vi "ConditionalUnsigned8.vi"(11 "?":u8) -> (2 "Value String":string, 3 "Stop?":bool)   [LabVIEW 2017]
doc: "Displays the value of the 8-bit unsigned integer numeric control and allows conditional breakpoints."
panel:
  in  "Tab Control":enum32{"Data   ", "Condition      "}(tab)
  out "Value":u8
  in  "Ls":u8
  in  "Gr":u8
  in  "Eq":u8
  in  "Ls":bool
  in  "Gr":bool
  in  "Eq":bool
  # "Pause if any of the following:"
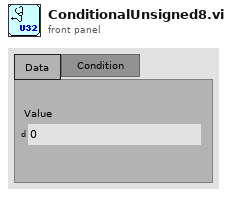
[diagram p1: front panel]
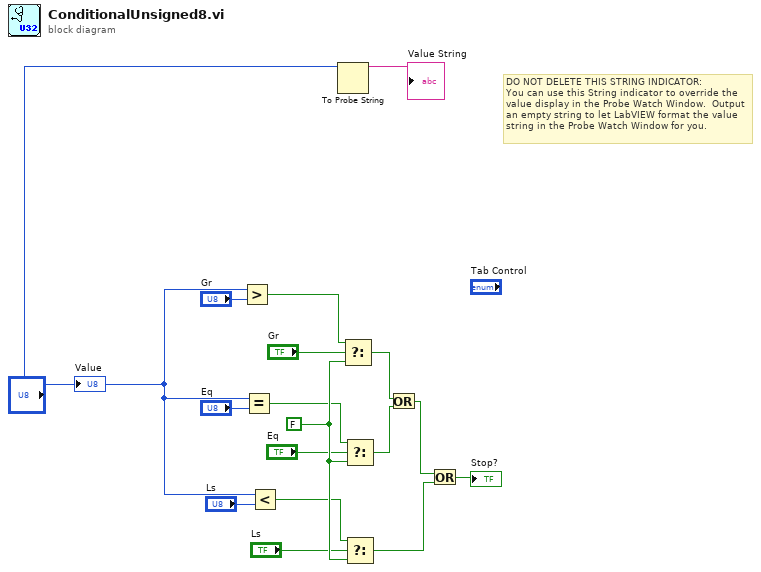
[diagram p0: block diagram]
diagram:
  w14 = FALSE ("f")
  # "DO NOT DELETE THIS STRING INDICATOR: \nYou can use this String indicator to override the value display in the Probe Watch Window.  Output an empty string to let LabVIEW format the value string in the Probe Watch Window for you."
  n1 = Greater?(x="?", y="Gr") -> (0:w2:bool)
  n2 = Equal?(x="?", y="Eq") -> (x = y?=w11:bool)
  n3 = Less?(x="?", y="Ls") -> (x < y?=w4:bool)
  n4 = To Probe String(7:"?") -> (3:→"Value String":string)  [unwired: 2 in, 1 out]
  n5 = Select(t=w2, s="Gr", f=w14) -> (s? t:f=w8:bool)
  n6 = Select(t=w11, s="Eq", f=w14) -> (s? t:f=w7:bool)
  n7 = Select(t=w4, s="Ls", f=w14) -> (s? t:f=w5:bool)
  n8 = Or(x=w8, y=w7) -> (x .or. y?=w6:bool)
  n9 = Or(x=w6, y=w5) -> (x .or. y?=→"Stop?":bool)
  "Value" <- "?"
